vi "ziPollDataExDemodTime.vi"(8 "error in":errorcluster, 9 "recording time (1) [s]":dbl=1.0, 10 "SubscribepathArray":string[](array[string])=["demods/0/sample"], 11 "Handle In":T2 {"Handle" format="0x%08x"; "Conn" format="0x%08x"}) -> (0 "error out":errorcluster, 2 "Demod Sample Out":T1[](array[typedef]) {"Aux In 1 (V)" format="%#_5p"; "Aux In 0 (V)" format="%#_5p"; "X (Vrms)" format="%#_5p"; "Y (Vrms)" format="%#_5p"; "Osc Phase (rad)" format="%#.3g"}, 3 "Handle Out":T2 {"Handle" format="0x%08x"; "Conn" format="0x%08x"})   [LabVIEW 2009, in "Zurich Instruments LabOne.lvlib"]
doc: "This vi polls <b>Demod data</b> from a previously subscriped demod path for a given <b>recording time</b>."
uses:
  <instrlib>/Zurich Instruments LabOne/Zurich Instruments LabOne.lvlib
  <instrlib>/Zurich Instruments LabOne/Public/ziTypeHandle.ctl
  <instrlib>/Zurich Instruments LabOne/Public/Data/ziTypeDemodSampleEx.ctl
  <instrlib>/Zurich Instruments LabOne/Public/Utility/ziTicksToS_vector.vi
  <instrlib>/Zurich Instruments LabOne/Public/Data/ziGetEventDemodSample.vi
panel:
  out "?":i32
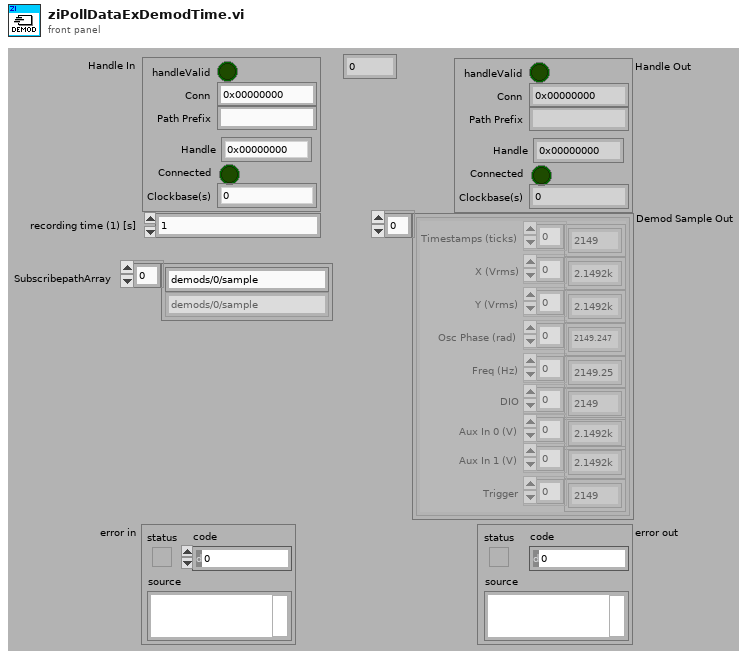
[diagram p1: front panel]
types:
  T1 = typedef "Zurich Instruments LabOne.lvlib/ziTypeDemodSampleEx.ctl" = cluster{"Timestamps (ticks)":u64[], "X (Vrms)":dbl[], "Y (Vrms)":dbl[], "Osc Phase (rad)":dbl[], "Freq (Hz)":dbl[], "DIO":u32[], "Aux In 0 (V)":dbl[], "Aux In 1 (V)":dbl[], "Trigger":u32[]}
  T2 = typedef "Zurich Instruments LabOne.lvlib/ziTypeHandle.ctl" = cluster{"handleValid":bool, "Conn":u64, "Path Prefix":string, "Handle":u64, "Connected":bool, "Clockbase(s)":dbl}
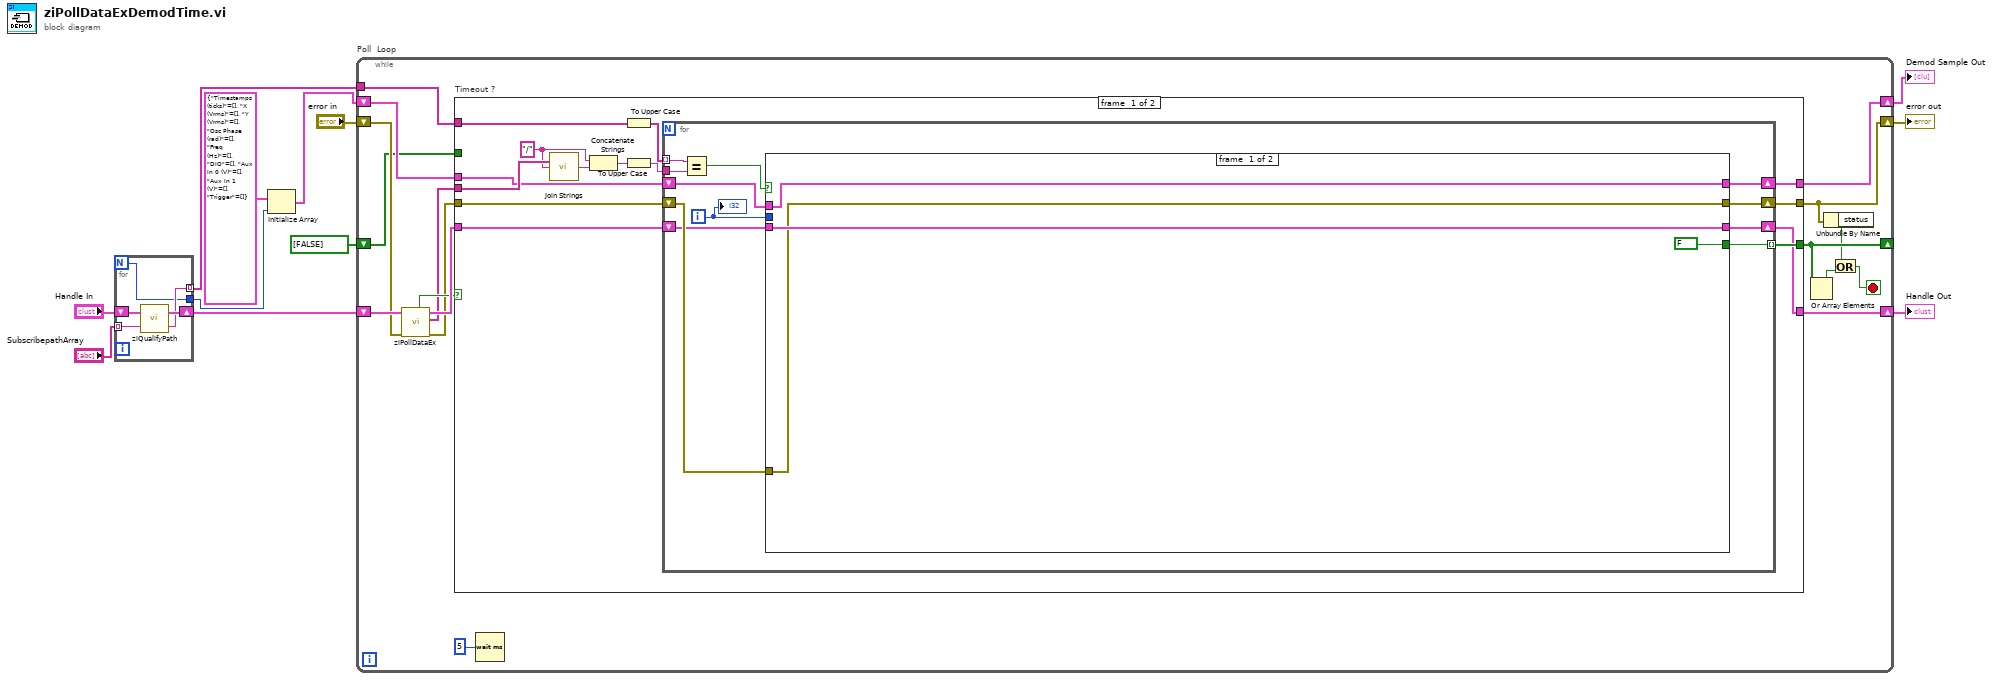
[diagram p0: block diagram]
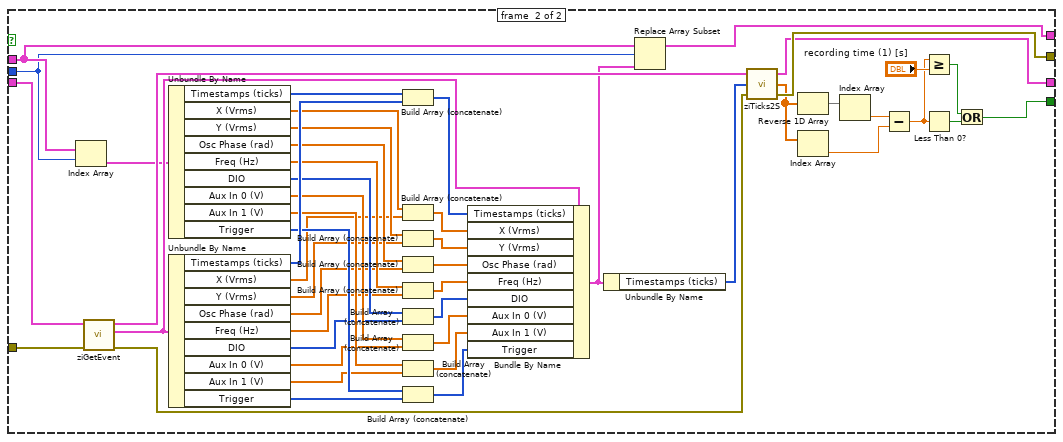
[diagram p2: hidden frame]
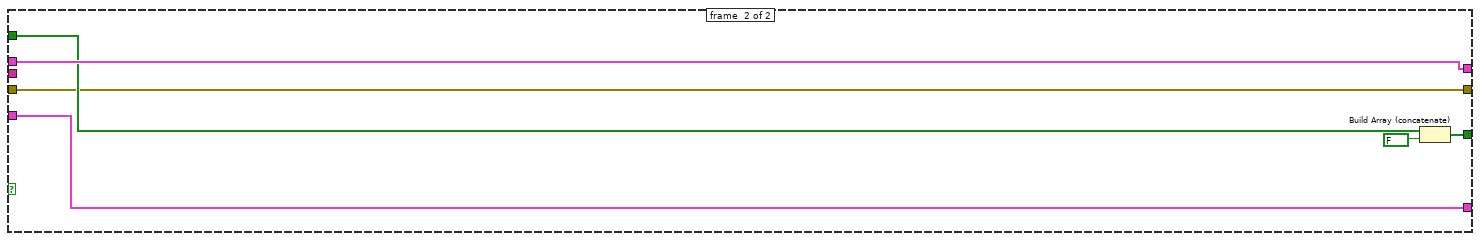
[diagram p3: hidden frame]
diagram:
  n1 = for {
    N -> [w13]
    tunnel: "SubscribepathArray" -> [w15] mode=indexing
    tunnel: [w14] -> w6 mode=indexing
    shift-right: [w16] -> w8
    shift-left: "Handle In" -> [w17]
    tunnel: [w13] -> w3
    n2 = call <instrlib>:"ziQualifyPath.vi"("Path In"=w15, "Handle In"=w17) -> ("Path Out"=w14:string, "Handle Out"=w16:T2)
  }
  n3 = Initialize Array(T1 {"Timestamps (ticks)"=[], "X (Vrms)"=[], "Y (Vrms)"=[], "Osc Phase (rad)"=[], "Freq (Hz)"=[], "DIO"=[], "Aux In 0 (V)"=[], "Aux In 1 (V)"=[], "Trigger"=[]} ("Demod Sample Out"), w3) -> (w2:T1[])
  n4 = while "Poll  Loop" {
    shift-right: [w24] -> w12
    shift-left: w8 -> [w29]
    shift-right: [w21] -> w11
    shift-left: "error in" -> [w28]
    tunnel: w6 -> [w27]
    shift-right: [w26] -> w5
    shift-left: w2 -> [w25]
    shift-right: [w22] -> _
    shift-left: bool[] [FALSE] -> [w23]
    stop <- w18 stop-if-true
    n5 = call <instrlib>:"ziPollDataEx.vi"("error in"=w28, "Handle In"=w29) -> ("error out"=w32:errorcluster, "PathArray"=w31:string[], "Handle Out"=w34:T2, "Timed Out"=w33:bool)  [unwired: 2 in, 4 out]
    n6 = case "Timeout ?" shown="False" w33 {
      tunnel: w34 -> [w37 w117]
      tunnel: w32 -> [w48 w113]
      tunnel: [w47 w113] -> w21
      tunnel: w31 -> [w45 _]
      tunnel: w27 -> [w41 _]
      tunnel: [w39 w115] -> w22
      tunnel: [w35 w118] -> w26
      tunnel: w25 -> [w38 w118]
      tunnel: [w36 w117] -> w24
      tunnel: w23 -> [_ w116]
      frame #0 {
        w44 = "/" ("Separator (,)")
        n7 = call <vilib>:"Join Strings.vi"("Separator (,)"=w44, "Strings In"=w45) -> ("String"=w46:string)  [unwired: 1 in]
        n8 = Concatenate Strings(w44, w46) -> (w40:string)
        n9 = To Upper Case(1:w41) -> (0:w42:string[])
        n10 = To Upper Case(1:w40) -> (0:w43:string)
        n11 = for {
          tunnel: w43 -> [w56]
          tunnel: w42 -> [w55] mode=indexing
          tunnel: [w54] -> w39 mode=indexing
          shift-right: [w57] -> w47
          shift-left: w48 -> [w58]
          shift-right: [w59] -> w36
          shift-left: w37 -> [w52]
          shift-right: [w51] -> w35
          shift-left: w38 -> [w50]
          i -> [w49]
          n12 = Equal?(x=w55, y=w56) -> (x = y?=w53:bool)
          n13 = case shown="True" w53 {
            tunnel: w52 -> [w63 w112]
            tunnel: [w63 w79] -> w59
            tunnel: w58 -> [w62 w111]
            tunnel: [w62 w80] -> w57
            tunnel: [FALSE w70] -> w54
            tunnel: [w60 w68] -> w51
            tunnel: w50 -> [w60 w65]
            tunnel: w49 -> [_ w64]
            frame #0 {
            }
            frame #1 {
              n14 = Index Array(array=w65, index=w64) -> (element=w66:T1)
              n15 = call-poly <instrlib>:"ziGetEvent.vi"("Error In"=w111, "Handle In"=w112) -> ("Error Out"=w82:errorcluster, "Demod Sample Out"=w69:T1, "Handle Out"=w83:T2)  [unwired: 7 in]
              n16 = Unbundle By Name(w66) -> ("Timestamps (ticks)"=w110:u64[], "X (Vrms)"=w107:dbl[], "Y (Vrms)"=w106:dbl[], "Osc Phase (rad)"=w105:dbl[], "Freq (Hz)"=w104:dbl[], "DIO"=w99:u32[], "Aux In 0 (V)"=w98:dbl[], "Aux In 1 (V)"=w97:dbl[], "Trigger"=w96:u32[])
              n17 = Unbundle By Name(w69) -> ("Timestamps (ticks)"=w109:u64[], "X (Vrms)"=w91:dbl[], "Y (Vrms)"=w90:dbl[], "Osc Phase (rad)"=w89:dbl[], "Freq (Hz)"=w88:dbl[], "DIO"=w87:u32[], "Aux In 0 (V)"=w86:dbl[], "Aux In 1 (V)"=w85:dbl[], "Trigger"=w84:u32[])
              n18 = Build Array (concatenate)(w110, w109) -> (w108:u64[])
              n19 = Build Array (concatenate)(w107, w91) -> (w103:dbl[])
              n20 = Build Array (concatenate)(w106, w90) -> (w102:dbl[])
              n21 = Build Array (concatenate)(w105, w89) -> (w101:dbl[])
              n22 = Build Array (concatenate)(w104, w88) -> (w100:dbl[])
              n23 = Build Array (concatenate)(w99, w87) -> (w95:u32[])
              n24 = Build Array (concatenate)(w98, w86) -> (w94:dbl[])
              n25 = Build Array (concatenate)(w97, w85) -> (w93:dbl[])
              n26 = Build Array (concatenate)(w96, w84) -> (w92:u32[])
              n27 = Bundle By Name(cluster=w69, "Timestamps (ticks)"=w108, "X (Vrms)"=w103, "Y (Vrms)"=w102, "Osc Phase (rad)"=w101, "Freq (Hz)"=w100, "DIO"=w95, "Aux In 0 (V)"=w94, "Aux In 1 (V)"=w93, "Trigger"=w92) -> (w67:T1)
              n28 = Unbundle By Name(w67) -> ("Timestamps (ticks)"=w81:u64[])
              n29 = Replace Array Subset(array=w65, new element=w67, index=w64) -> (w68:T1[])
              n30 = call-poly <instrlib>:"ziTicks2S.vi"("Error In"=w82, "Timestamp (ticks)"=w81, "Handle In"=w83) -> ("Error Out"=w80:errorcluster, "Timestamp(s)"=w77:dbl[], "Handle Out"=w79:T2)
              n31 = Reverse 1D Array(array=w77) -> (reversed array=w78:dbl[])
              n32 = Index Array(array=w77) -> (element=w75:dbl)  [unwired: 1 in]
              n33 = Index Array(array=w78) -> (element=w76:dbl)  [unwired: 1 in]
              n34 = Subtract(x=w76, y=w75) -> (x-y=w72:dbl)
              n35 = Greater Or Equal?(x=w72, y="recording time (1) [s]") -> (x >= y?=w71:bool)
              n36 = Less Than 0?(x=w72) -> (x < 0?=w73:bool)
              n37 = Or(x=w71, y=w73) -> (x .or. y?=w70:bool)
            }
          }
          "?" <- w49
        }
      }
      frame #1 {
        n38 = Build Array (concatenate)(w116, FALSE) -> (w115:bool[])
      }
    }
    n39 = Wait (ms)(milliseconds to wait=u32 5) -> ()  [unwired: 1 out]
    n40 = Or Array Elements(Boolean array=w22) -> (logical OR=w20:bool)
    n41 = Unbundle By Name(w21) -> ("status"=w19:bool)
    n42 = Or(x=w19, y=w20) -> (x .or. y?=w18:bool)
  }
  "Handle Out" <- w12
  "error out" <- w11
  "Demod Sample Out" <- w5
